vi "JL_Next Dryness Or Temp Option.vi"(0 "Current Option":u8 format="%x", 5 "Allowables":u8 format="%x", 7 "Default":u8 format="%x") -> (4 "Fail":bool, 6 "Pass":bool, 8 "Report Text":string, 10 "Next Option":u8 format="%x", 15 "Next Tone":T1)   [LabVIEW 2016]
uses:
  Type Defs/JL_Tones.ctl
panel:
  # "All integers are hex"
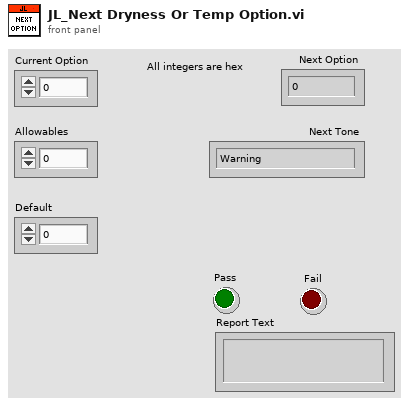
[diagram p1: front panel]
types:
  T1 = typedef "JL_Tones.ctl" = enum16{"Warning", "PowerUp", "PowerDown", "IncreaseSound", "DecreaseSound", "Ok", "OkVolumeKey", "Unavailable", "KnobTurn", "Notification1", "Notification2", "Notification3", "NotificationIntro", "NotificationEnd", "FeatureOn", "FeatureOff", "HoldOn", "HoldOnVolumeKey", "HoldOff", "Max", "None"}
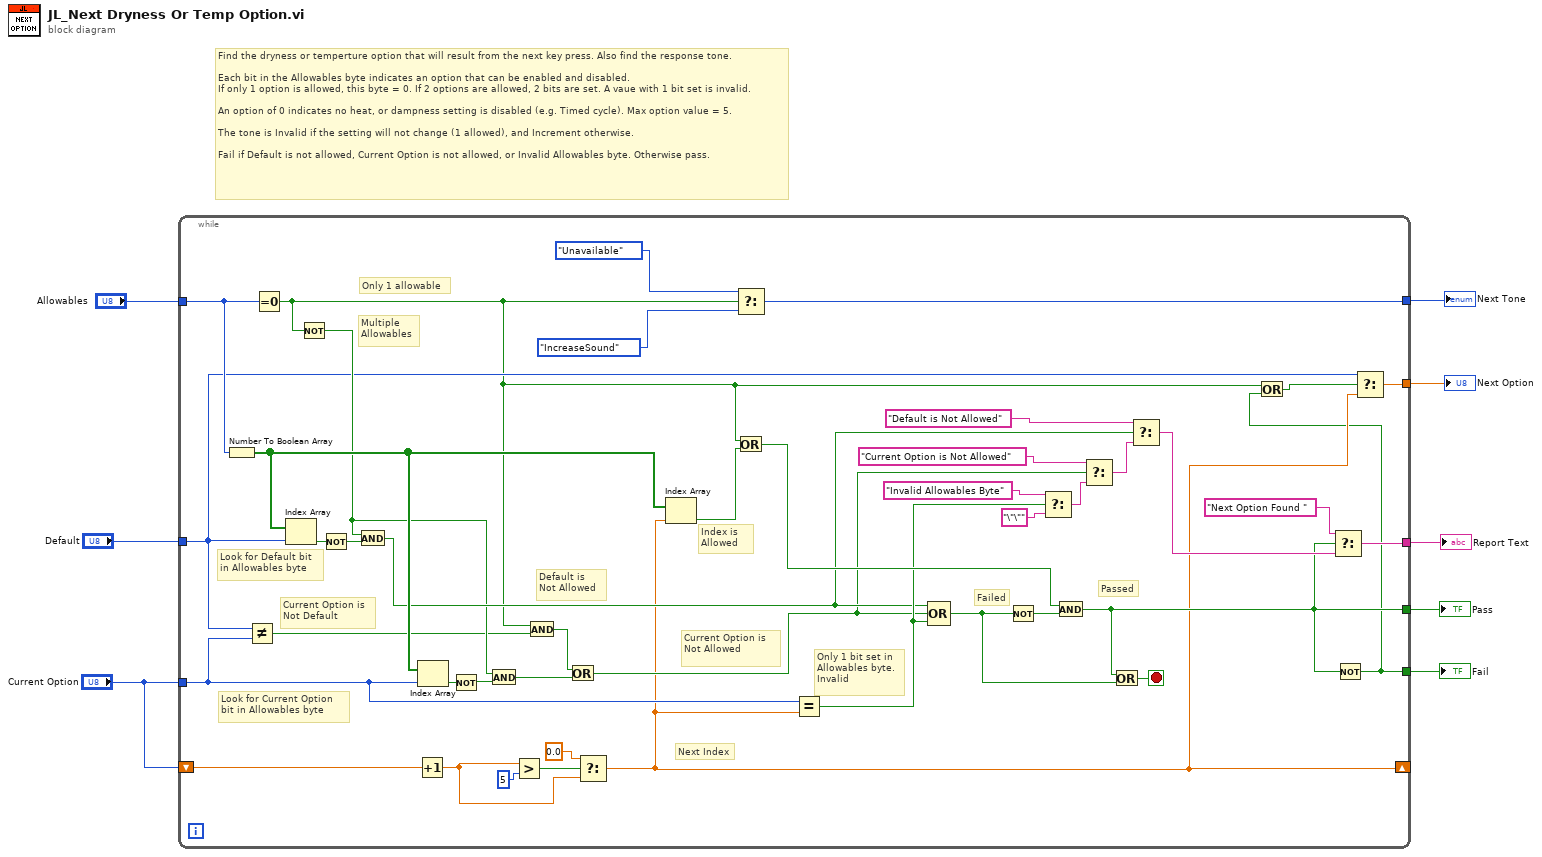
[diagram p0: block diagram]
diagram:
  # "Find the dryness or temperture option that will result from the next key press. Also find the response tone.\n\nEach bit in the Allowables byte indicates an option that can be enabled and disabled.\nIf only 1 option is allowed, this byte = 0. If 2 options are allowed, 2 bits are set. A vaue with 1 bit set is invalid.\n\nAn option of 0 indicates no heat, or dampness setting is disabled (e.g. Timed cycle). Max option value = 5.\n\nThe tone is Invalid if the setting will not change (1 allowed), and Increment otherwise.\n\nFail if Default is not allowed, Current Option is not allowed, or Invalid Allowables byte. Otherwise pass."
  n1 = while {
    tunnel: [w51] -> w1
    tunnel: "Allowables" -> [w50]
    tunnel: "Current Option" -> [w18]
    tunnel: "Default" -> [w19]
    shift-right: [w12] -> _
    shift-left: "Current Option" -> [w49]
    tunnel: [w43] -> w5
    tunnel: [w15] -> w4
    tunnel: [w37] -> w3
    tunnel: [w9] -> w2
    stop <- w39 stop-if-true
    # "Current Option is\nNot Default"
    # "Look for Current Option\nbit in Allowables byte"
    # "Look for Default bit\nin Allowables byte"
    # "Multiple\nAllowables"
    # "Passed"
    # "Failed"
    # "Only 1 bit set in\nAllowables byte.\nInvalid"
    # "Next Index"
    # "Index is Allowed"
    # "Default is\nNot Allowed"
    # "Current Option is Not Allowed"
    # "Only 1 allowable"
    n2 = Number To Boolean Array(number=w50) -> (Boolean array=w44:bool[])
    n3 = Not Equal?(x=w19, y=w18) -> (x != y?=w20:bool)
    n4 = Equal To 0?(x=w50) -> (x = 0?=w11:bool)
    n5 = Index Array(array=w44, index=w19) -> (element=w42:bool)
    n6 = Not(x=w11) -> (.not. x?=w22:bool)
    n7 = Not(x=w42) -> (.not. x?=w25:bool)
    n8 = And(x=w22, y=w25) -> (x .and. y?=w24:bool)
    n9 = Increment(x=w49) -> (x+1=w45:dbl)
    n10 = Index Array(array=w44, index=w18) -> (element=w41:bool)
    n11 = Not(x=w41) -> (.not. x?=w23:bool)
    n12 = And(x=w22, y=w23) -> (x .and. y?=w21:bool)
    n13 = Greater?(x=w45, y=u8 5) -> (0:w47:bool)
    n14 = And(x=w11, y=w20) -> (x .and. y?=w16:bool)
    n15 = Or(x=w16, y=w21) -> (x .or. y?=w17:bool)
    n16 = Select(t=0.0, s=w47, f=w45) -> (s? t:f=w12:dbl)
    n17 = Index Array(array=w44, index=w12) -> (element=w29:bool)
    n18 = Select(t=JL_Tones."Unavailable" ("Increase Tone"), s=w11, f=JL_Tones."IncreaseSound" ("Increase Tone")) -> (s? t:f=w51:T1)
    n19 = Or(x=w11, y=w29) -> (x .or. y?=w28:bool)
    n20 = Equal?(x=w18, y=w12) -> (x = y?=w27:bool)
    n21 = Compound Arithmetic op=OR(w24, w17, w27) -> (w38:bool)
    n22 = Not(x=w38) -> (.not. x?=w40:bool)
    n23 = Select(t="Invalid Allowables Byte" ("string"), s=w27, f="\"\"") -> (s? t:f=w31:string)
    n24 = And(x=w28, y=w40) -> (x .and. y?=w15:bool)
    n25 = Select(t="Current Option is Not Allowed" ("string"), s=w17, f=w31) -> (s? t:f=w33:string)
    n26 = Or(x=w15, y=w38) -> (x .or. y?=w39:bool)
    n27 = Select(t="Default is Not Allowed" ("string"), s=w24, f=w33) -> (s? t:f=w35:string)
    n28 = Select(t="Next Option Found " ("string"), s=w15, f=w35) -> (s? t:f=w37:string)
    n29 = Not(x=w15) -> (.not. x?=w9:bool)
    n30 = Or(x=w11, y=w9) -> (x .or. y?=w10:bool)
    n31 = Select(t=w19, s=w10, f=w12) -> (s? t:f=w43:dbl)
  }
  "Pass" <- w4
  "Report Text" <- w3
  "Next Option" <- w5
  "Fail" <- w2
  "Next Tone" <- w1
